vi "Compute Gradient 64f.vi"(8 "Error In":errorcluster, 10 "Input":T1 {"Dimension"."Width" min=1; "Dimension"."Height" min=1; "Dimension"."Depth" min=1}, 11 "Gradient Object":T6 {"Z"."Dimension"."Width" min=1; "Z"."Dimension"."Height" min=1; "Z"."Dimension"."Depth" min=1; "Y"."Dimension"."Width" min=1; "Y"."Dimension"."Height" min=1; "Y"."Dimension"."Depth" min=1; "X"."Dimension"."Width" min=1; "X"."Dimension"."Height" min=1; "X"."Dimension"."Depth" min=1}) -> (0 "Error Out":errorcluster, 1 "Z":T1 {"Dimension"."Width" min=1; "Dimension"."Height" min=1; "Dimension"."Depth" min=1}, 2 "Y":T1 {"Dimension"."Width" min=1; "Dimension"."Height" min=1; "Dimension"."Depth" min=1}, 3 "X":T1 {"Dimension"."Width" min=1; "Dimension"."Height" min=1; "Dimension"."Depth" min=1}, 4 "Time in ms":dbl)   [LabVIEW 2012, in "OpenCLV x64.lvlib"]
doc: "Computes the Gradient based on already created Gradient Object. The dimensions of the input array <b>must</b> match the size of the dimension used to define the Gradient Object."
uses:
  OpenCLV x64.lvlib
  Controls/Gradient Object.ctl
  Controls/Program Handle.ctl
  Controls/Device ID.ctl
  Controls/Memory Object.ctl
  Controls/Memory ID.ctl
  User Controls/Array Dimensions.ctl
  Controls/Memory Type.ctl
  Set Kernel Arguments/Set Kernel Arguments Memory Object.vi
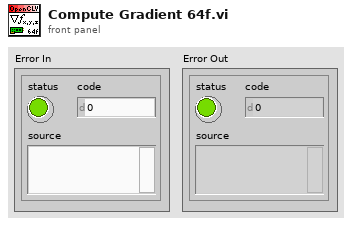
[diagram p1: front panel]
types:
  T1 = typedef "OpenCLV x64.lvlib/Memory Object.ctl" = cluster{"Device ID":T2, "Memeroy ID":T3, "Dimension":T4, "Memory Type":T5}
  T2 = typedef "OpenCLV x64.lvlib/Device ID.ctl" = u64
  T3 = typedef "OpenCLV x64.lvlib/Memory ID.ctl" = u64
  T4 = typedef "Array Dimensions.ctl" = cluster{"Depth":u64, "Height":u64, "Width":u64}
  T5 = typedef "OpenCLV x64.lvlib/Memory Type.ctl" = enum16{"32f", "u8", "i8", "u16", "i16", "u32", "i32", "64f"}
  T6 = typedef "OpenCLV x64.lvlib/Gradient Object.ctl" = cluster{"Program Handle":T7, "Device Out":T2, "X":T1, "Y":T1, "Z":T1}
  T7 = typedef "OpenCLV x64.lvlib/Program Handle.ctl" = u64
  T8 = typedef "OpenCLV x64.lvlib/Kernel Handle.ctl" = u64
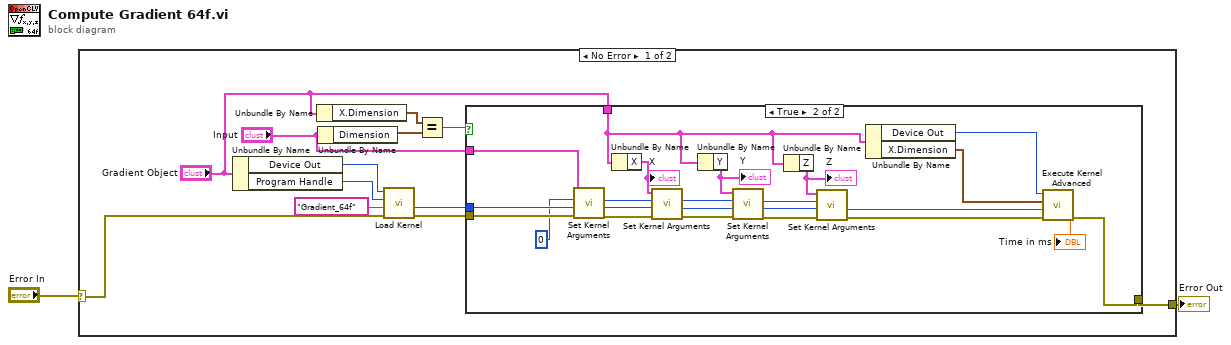
[diagram p0: block diagram]
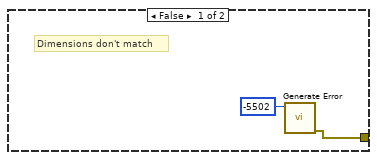
[diagram p2: hidden frame]
diagram:
  n1 = case shown="No Error" "Error In" {
    selector: "Error In" -> [w14 w40]
    tunnel: [w8 w40] -> w1
    frame No Error {
      n2 = Unbundle By Name("Gradient Object") -> ("Device Out"=w12:T2, "Program Handle"=w13:T7)
      n3 = Unbundle By Name("Gradient Object") -> ("X.Dimension"=w6:T4)
      n4 = Unbundle By Name("Input") -> ("Dimension"=w5:T4)
      n5 = call "Load Kernel.vi"("Error In"=w14, "Kernel Name"="Gradient_64f", "Program Handle"=w13, "Device In"=w12) -> ("Error Out"=w10:errorcluster, "Kernel Handle"=w9:T8)  [unwired: 4 in, 2 out]
      n6 = Equal?(x=w6, y=w5) -> (x = y?=w4:bool)
      n7 = case shown="True" w4 {
        tunnel: w10 -> [_ w39]
        tunnel: w9 -> [_ w38]
        tunnel: [w16 w18] -> w8
        tunnel: "Gradient Object" -> [_ w20]
        tunnel: "Input" -> [_ w19]
        frame False {
          # "Dimensions don't match"
          n8 = call "Generate Error.vi"("Error"=-5502) -> ("error out"=w16:errorcluster)  [unwired: 10 in]
        }
        frame True {
          n9 = call-poly "Set Kernel Arguments.vi"("Error In"=w39, "Kernel Handle"=w38, "Argument Number"=0, "Memory Object"=w19) -> ("Error Out"=w34:errorcluster, "Kernel Handle out"=w35:T8, "Auto Inc Arugment Number"=w36:i32)  [unwired: 5 in]
          n10 = Unbundle By Name(w20) -> ("X"=w27:T1)
          "X" <- w27
          n11 = call-poly "Set Kernel Arguments.vi"("Error In"=w34, "Kernel Handle"=w35, "Argument Number"=w36, "Memory Object"=w27) -> ("Error Out"=w33:errorcluster, "Kernel Handle out"=w32:T8, "Auto Inc Arugment Number"=w31:i32)  [unwired: 5 in]
          n12 = Unbundle By Name(w20) -> ("Y"=w26:T1)
          "Y" <- w26
          n13 = call-poly "Set Kernel Arguments.vi"("Error In"=w33, "Kernel Handle"=w32, "Argument Number"=w31, "Memory Object"=w26) -> ("Error Out"=w30:errorcluster, "Kernel Handle out"=w29:T8, "Auto Inc Arugment Number"=w28:i32)  [unwired: 5 in]
          n14 = Unbundle By Name(w20) -> ("Z"=w25:T1)
          "Z" <- w25
          n15 = call-poly "Set Kernel Arguments.vi"("Error In"=w30, "Kernel Handle"=w29, "Argument Number"=w28, "Memory Object"=w25) -> ("Error Out"=w24:errorcluster, "Kernel Handle out"=w23:T8)  [unwired: 5 in, 1 out]
          n16 = Unbundle By Name(w20) -> ("Device Out"=w22:T2, "X.Dimension"=w17:T4)
          n17 = call "Execute Kernel Advanced.vi"("Error In"=w24, "Kernel Handle"=w23, "Thread Dimensions"=w17, "Device In"=w22) -> ("Error Out"=w18:errorcluster, "Time in ms"=→"Time in ms":dbl)  [unwired: 4 in, 2 out]
        }
      }
    }
    frame Error {
    }
  }
  "Error Out" <- w1
